vi "module permission to classification.vi"(11 "display permissions":T1) -> (3 "channel classification":T2)   [LabVIEW 2015, in "PID Module configuration.lvclass"]
doc: "Converts from the 'display permissions' type-def to the 'channel classification' type-def."
uses:
  PID Module configuration.lvclass
  <vilib>/NI/Tag Bus Module Framework/channel/channel classification.ctl
  permissions.ctl
  <vilib>/NI/Tag Bus Module Framework/channel/TBM channel.lvclass
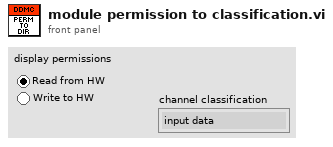
[diagram p1: front panel]
types:
  T1 = typedef "PID Module configuration.lvclass/permissions.ctl" = enum32{"Read from HW", "Write to HW"}
  T2 = typedef "TBM channel.lvclass/channel classification.ctl" = enum16{"input data", "output data", "processing parameter", "processing result"}
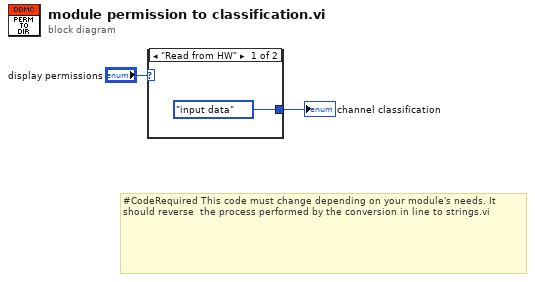
[diagram p0: block diagram]
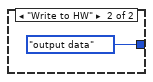
[diagram p2: hidden frame]
diagram:
  # "#CodeRequired This code must change depending on your module's needs. It should reverse  the process performed by the conversion in line to strings.vi"
  n1 = case shown="\"Read from HW\"" "display permissions" {
    tunnel: [channel_classification."input data" ("channel classification") channel_classification."output data" ("channel classification")] -> w2
    frame "Read from HW" {
    }
    frame "Write to HW" {
    }
  }
  "channel classification" <- w2
